vi "Enqueue-Background Imaging data.vi"(8 "error in (no error)":errorcluster, 9 "Element to queue":T1, 10 "Logging queue element":T3={"Imaging Protocol"=enum."Live Imaging", "Number of Trials"=0, "Frame Size"=512, "# Averaged frames"=0, "Dwell time (us)"=0.0, "Index of Z-plane"=0, "Timelapse?"=FALSE, "Logging process is active"=FALSE, "Speed logging enabled"=FALSE, "tdms file ref"=refnum, "path"=path "", "Trial Number"=0, "Expected # points acquired"=FALSE, "Manually stopped"=FALSE, "Ch0 data"=[], "Ch1 data"=[], "Ref Data"=[], "Last trial"=FALSE, "Ref Dwell time (us)"=0.0, "# Ref Averaged frames"=0, "Ref X Length"=0, "Ref Y Length"=0, "Points acquired"={"Ch0 last trial"=0, "Ch1 last trial"=0, "All trials"=0}} {"Ref Dwell time (us)" format="%#.6g"; "Frame Size" items=["100X100"=100, "128X128"=128, "200X200"=200, "256X256"=256, "512X512"=512, "1024x1024"=1024, "2048x2048"=2048]; "Dwell time (us)" format="%#.6g"}, 11 "Live graph data queue in":T7) -> (0 "error out":errorcluster, 3 "Live graph data queue":T7)   [LabVIEW 2017]
uses:
  Typedefs/Live graph data queue ref.ctl
  Live graphs queue/Typedefs/Live imaging queue element.ctl
  <vilib>/vision/Image Controls.llb/IMAQ Image.ctl
  Typedefs/Logging queue element.ctl
  Typedefs/Imaging Protocols enum.ctl
  Typedefs/Frame Size.ctl
  Typedefs/Acquired points count.ctl
  Typedefs/Read Write Enum.ctl
panel:
  # "SUBROUTINE VI"
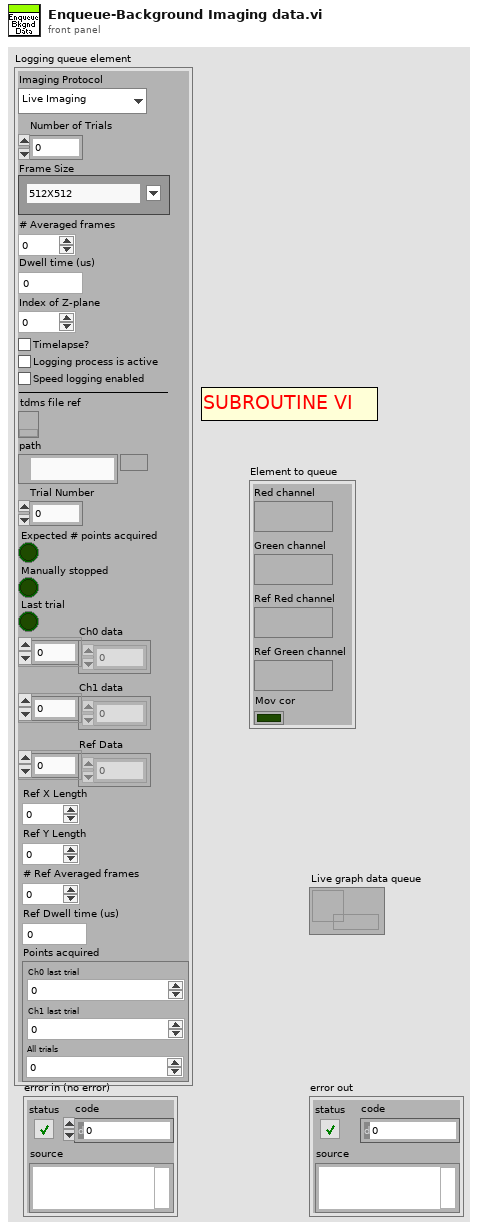
[diagram p1: front panel]
types:
  T1 = typedef "Live imaging queue element.ctl" = cluster{"Red channel":T2, "Green channel":T2, "Ref Red channel":T2, "Ref Green channel":T2, "Mov cor":bool}
  T2 = typedef "IMAQ Image.ctl" = refnum<image>
  T3 = typedef "Logging queue element.ctl" = cluster{"Imaging Protocol":T4, "Number of Trials":u16, "Frame Size":T5, "# Averaged frames":u16, "Dwell time (us)":dbl, "Index of Z-plane":i32, "Timelapse?":bool, "Logging process is active":bool, "Speed logging enabled":bool, "tdms file ref":refnum<k34>, "path":path, "Trial Number":i32, "Expected # points acquired":bool, "Manually stopped":bool, "Ch0 data":u32[], "Ch1 data":u32[], "Ref Data":u32[], "Last trial":bool, "Ref Dwell time (us)":dbl, "# Ref Averaged frames":u16, "Ref X Length":u16, "Ref Y Length":u16, "Points acquired":T6}
  T4 = typedef "Imaging Protocols enum.ctl" = enum16{"AOL Z-Stack", "Motor Z Stack", "Functional Acquisition", "Single Plane Acquisition", "Volume Acquisition", "Live Imaging", "Live Plane Imaging", "Live Volume Imaging"}
  T5 = typedef "Frame Size.ctl" = u16
  T6 = typedef "Acquired points count.ctl" = cluster{"Ch0 last trial":u64, "Ch1 last trial":u64, "All trials":u64}
  T7 = typedef "Live graph data queue ref.ctl" = refnum<queue>
  T8 = typedef "Read Write Enum.ctl" = enum16{"Read", "Write"}
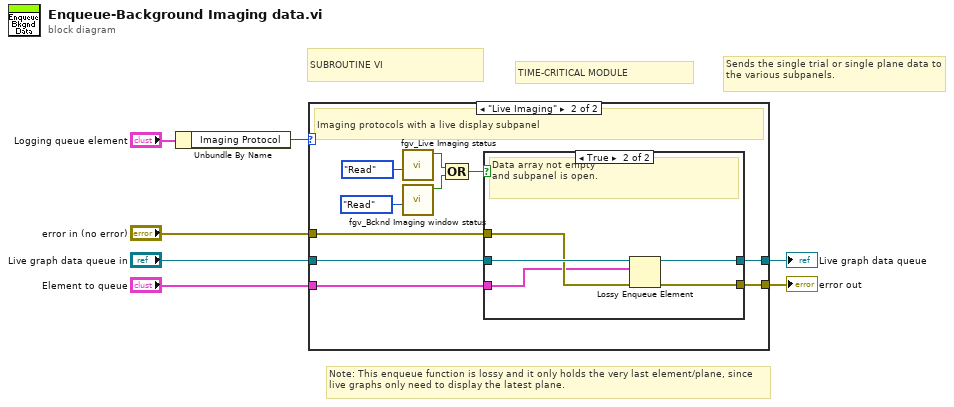
[diagram p0: block diagram]
diagram:
  # "TIME-CRITICAL MODULE"
  # "SUBROUTINE VI"
  # "Note: This enqueue function is lossy and it only holds the very last element/plane, since live graphs only need to display the latest plane."
  # "Sends the single trial or single plane data to the various subpanels."
  n1 = Unbundle By Name("Logging queue element") -> ("Imaging Protocol"=w2:T4)
  n2 = case shown="\"Live Imaging\"" w2 {
    tunnel: "error in (no error)" -> [w8 w19]
    tunnel: [w8 w18] -> w6
    tunnel: "Live graph data queue in" -> [w9 w17]
    tunnel: [w9 w16] -> w4
    tunnel: "Element to queue" -> [_ w15]
    frame Default {
      # "Imaging protocols without a live display subpanel."
    }
    frame "Live Imaging" {
      # "Imaging protocols with a live display subpanel"
      n3 = call "fgv_Live Imaging status.vi"("Function"=Read_Write_Enum."Read") -> ("Live Imaging?"=w13:bool)  [unwired: 9 in, 1 out]
      n4 = call "fgv_Bcknd Imaging window status.vi"("Function"=Read_Write_Enum."Read") -> ("Background MovCor window is open"=w10:bool)  [unwired: 9 in, 1 out]
      n5 = Compound Arithmetic op=OR(w13, w10) -> (w12:bool)
      n6 = case shown="True" w12 {
        tunnel: [w20 w26] -> w18
        tunnel: [w21 w25] -> w16
        tunnel: w17 -> [w21 w24]
        tunnel: w19 -> [w20 w23]
        tunnel: w15 -> [_ w22]
        frame False {
          # "Empty data array"
        }
        frame True {
          # "Data array not empty\nand subpanel is open."
          n7 = Lossy Enqueue Element(queue=w24, element=w22, error in (no error)=w23) -> (queue out=w25:T7, error out=w26:errorcluster)  [unwired: 2 out]
        }
      }
    }
  }
  "error out" <- w6
  "Live graph data queue" <- w4
